vi "Generate exported time series image path.vi"(7 "Channel":enum16{"Green", "Red"}(ring)=enum."Red", 9 "Minimum Width (4)":i16=4, 10 "FOR loop iteration":i32, 11 "Folder path":path) -> (3 "File path":path)   [LabVIEW 2020]
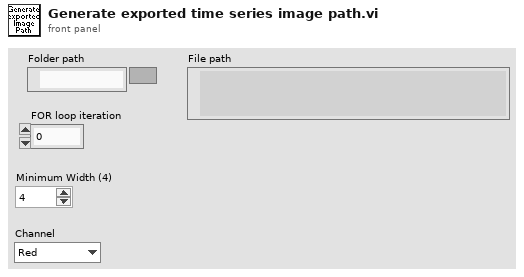
[diagram p1: front panel]
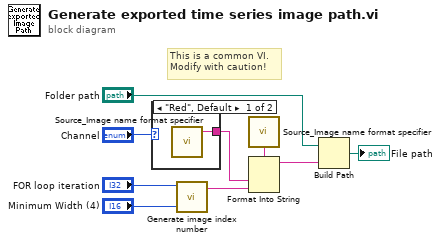
[diagram p0: block diagram]
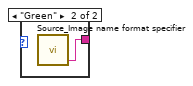
[diagram p2: hidden frame]
diagram:
  # "This is a common VI.\nModify with caution!"
  n1 = case shown="\"Red\", Default" "Channel" {
    tunnel: [w10 w11] -> w4
    frame "Red", Default {
      n2 = call "Source_Image name format specifier.vi"() -> ("Red channel name"=w10:string)  [unwired: 5 in, 2 out]
    }
    frame "Green" {
      n3 = call "Source_Image name format specifier.vi"() -> ("Green channel name"=w11:string)  [unwired: 5 in, 2 out]
    }
  }
  n4 = call "Generate image index number.vi"("Minimum Width (4)"="Minimum Width (4)", "FOR loop iteration or existing number of files"="FOR loop iteration") -> ("Number in string representation (padded with zeroes)"=w3:string)  [unwired: 9 in]
  n5 = call "Source_Image name format specifier.vi"() -> ("Z-Stack Image name format specifier"=w5:string)  [unwired: 5 in, 2 out]
  n6 = Format Into String(format string=w5, w4, w3) -> (resulting string=w6:string)  [unwired: 2 in, 1 out]
  n7 = Build Path(base path="Folder path", name or relative path=w6) -> (appended path=→"File path":path)
